vi "Units_MillisecondsToSeconds.vi"(10 "Milliseconds":dbl) -> (2 "Seconds":dbl)   [LabVIEW 2019, in "Trajectory_Library.lvlib"]
doc: "Convert a value from milliseoncds to seconds\n\nInputs: \n - Milliseconds\n\nOutputs:\n - Seconds"
uses:
  Trajectory_Library.lvlib
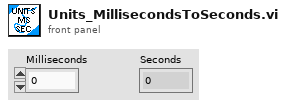
[diagram p1: front panel]
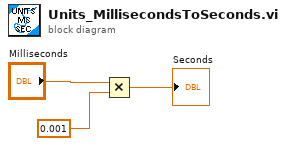
[diagram p0: block diagram]
diagram:
  n1 = Multiply(x="Milliseconds", y=0.001) -> (x*y=→"Seconds":dbl)
